vi "Command Rotate Ninety About Tote.vi"(2 "Input Robot System Funtions":T1, 3 "Cmd Parameter 1":dbl, 4 "Cmd Parameter 2":dbl, 5 "Startup":bool) -> (0 "Output Robot System Functions":T1, 1 "Completed":bool=TRUE)   [LabVIEW 2014]
uses:
  Subsystems VIs/Robot Commands.ctl
  Command Execution State.ctl
  Global Variables/Sensor Data (Edited).vi
  Global Variables/Settings.vi
panel:
  in  "Robot Twist Y":dbl=-19.0 format="%#_13g"
  in  "Robot Twist X":dbl=8.0 format="%#_13g"
  out "PID Tracking":cluster{"Goal Wheel Position":dbl, dbl}(graph)={"Goal Wheel Position"=0.0, -90.17571233858979}
  # "Sample robot\ncontrol output.\nReplace with \nactual teleop \ncontrol signal \nstructure."
  # "Field Centric"
  # "Field Centric"
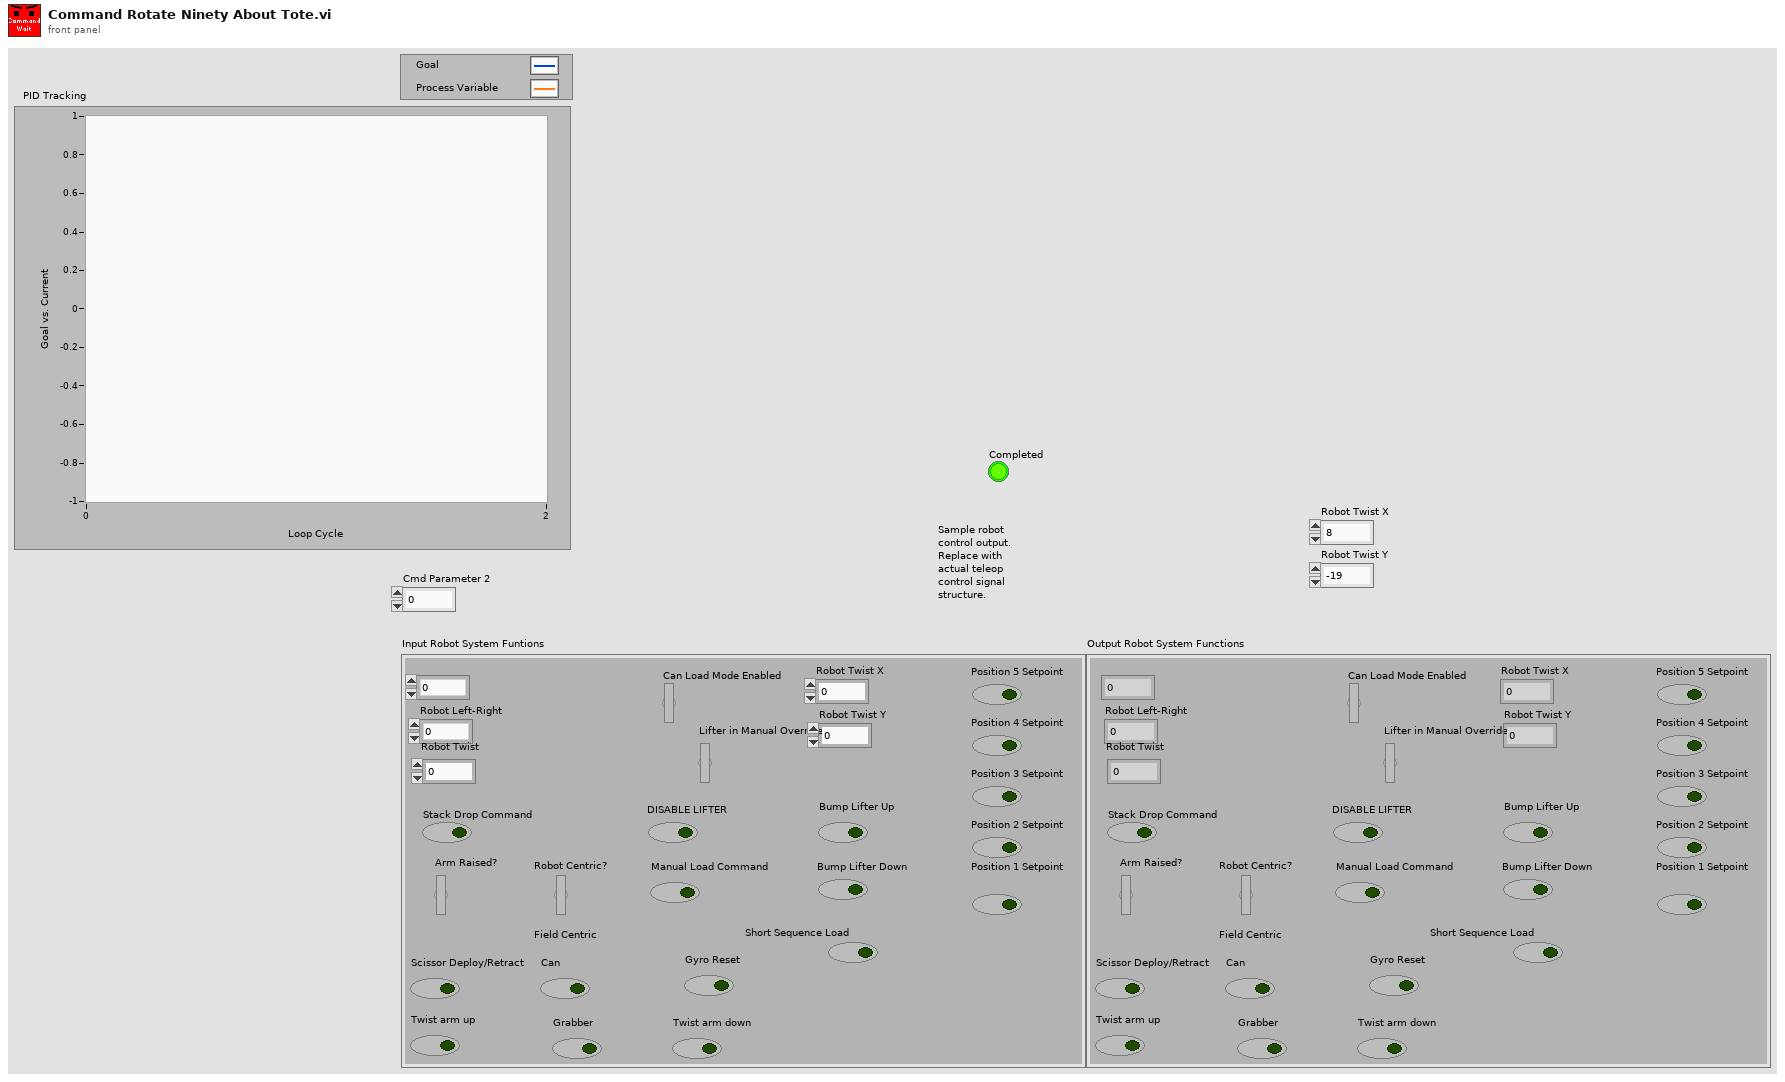
[diagram p1: front panel]
types:
  T1 = typedef "Robot Commands.ctl" = cluster{"Robot Forward-Reverse":dbl, "Robot Left-Right":dbl, "Robot Twist":dbl, "Can Load Mode Enabled":bool, "Lifter in Manual Override?":bool, "Stack Drop Command":bool, "Arm Raised?":bool, "DISABLE LIFTER":bool, "Position 1 Setpoint":bool, "Position 2 Setpoint":bool, "Position 3 Setpoint":bool, "Position 4 Setpoint":bool, "Position 5 Setpoint":bool, "Bump Lifter Down":bool, "Bump Lifter Up":bool, "Manual Load Command":bool, "Robot Centric?":bool, "Scissor Deploy/Retract":bool, "Grabber":bool, "Can":bool, "Twist arm up":bool, "Gyro Reset":bool, "Twist arm down":bool, "Short Sequence Load":bool, "Robot Twist X":dbl, "Robot Twist Y":dbl}
  T2 = typedef "Command Execution State.ctl" = enum16{"Initialize", "Execute", "Finish"}
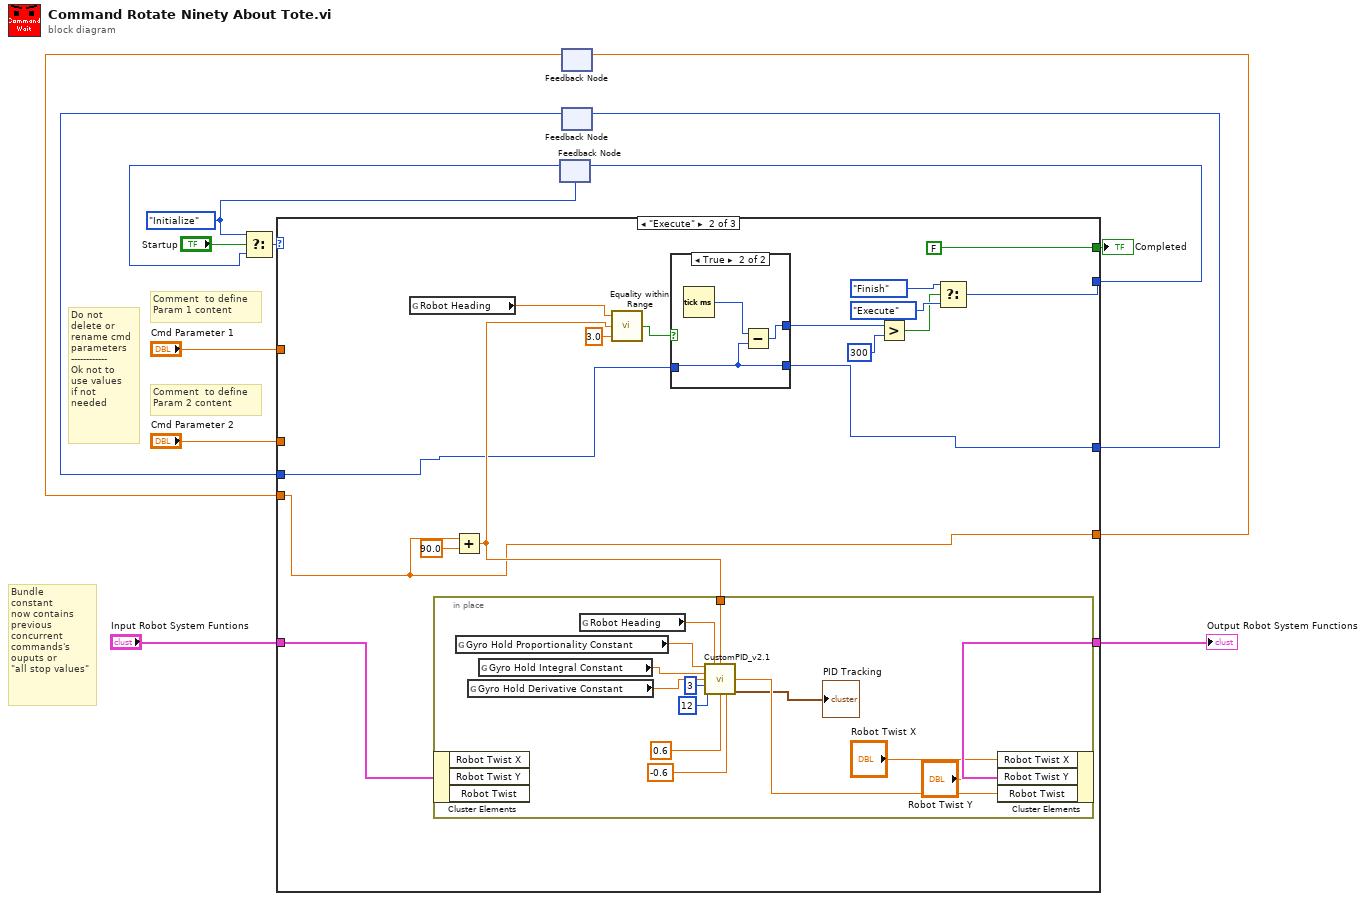
[diagram p0: block diagram]
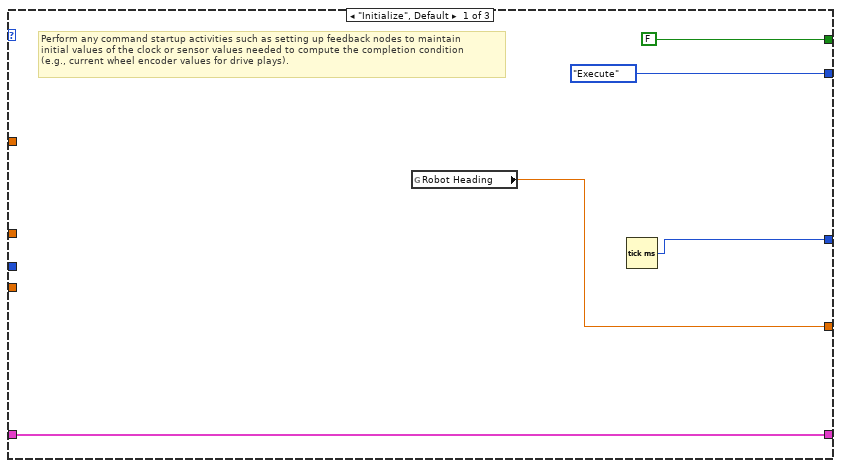
[diagram p2: hidden frame]
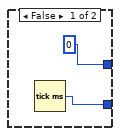
[diagram p3: hidden frame]
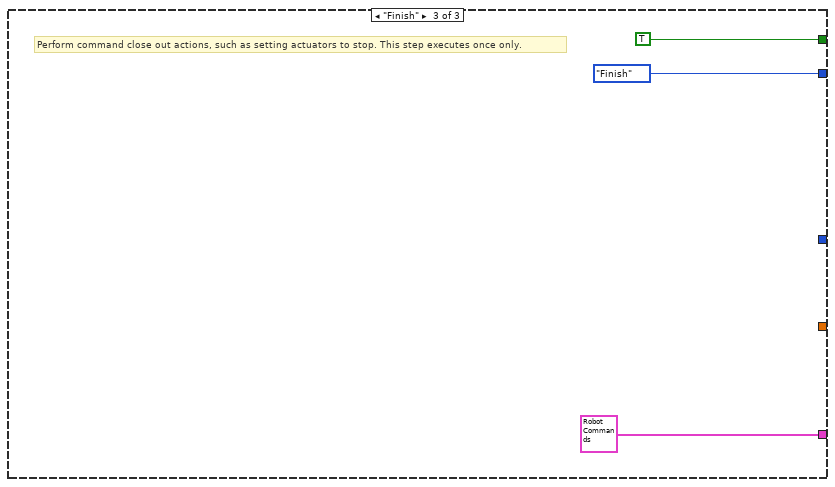
[diagram p4: hidden frame]
diagram:
  w9 = Command_Execution_State."Initialize" ("Play State")
  # "Bundle \nconstant\nnow contains\nprevious \nconcurrent\ncommands's\nouputs or\n\"all stop values\""
  # "Do not \ndelete or\nrename cmd\nparameters\n------------\nOk not to \nuse values\nif not \nneeded"
  # "Comment  to define\nParam 2 content"
  # "Comment  to define\nParam 1 content"
  n1 = feedback #1(w9) -> (w10:T2)
  n2 = Select(t=w9, s="Startup", f=w10) -> (s? t:f=w14:T2)
  n3 = feedback #2() -> (w3:dbl)  [unwired: 1 in]
  n4 = feedback #3() -> (w1:u32)  [unwired: 1 in]
  n5 = case shown="\"Execute\"" w14 {
    tunnel: [FALSE FALSE TRUE] -> w12
    tunnel: [Command_Execution_State."Execute" ("Play State") w21 Command_Execution_State."Finish" ("f")] -> w11
    tunnel: "Cmd Parameter 1" -> [_ _ _]
    tunnel: "Cmd Parameter 2" -> [_ _ _]
    tunnel: [w17 w25 T1 {"Robot Forward-Reverse"=0.0, "Robot Left-Right"=0.0, "Robot Twist"=0.0, "Can Load Mode Enabled"=FALSE, "Lifter in Manual Override?"=FALSE, "Stack Drop Command"=FALSE, "Arm Raised?"=FALSE, "DISABLE LIFTER"=FALSE, "Position 1 Setpoint"=FALSE, "Position 2 Setpoint"=FALSE, "Position 3 Setpoint"=FALSE, "Position 4 Setpoint"=FALSE, "Position 5 Setpoint"=FALSE, "Bump Lifter Down"=FALSE, "Bump Lifter Up"=FALSE, "Manual Load Command"=FALSE, "Robot Centric?"=FALSE, "Scissor Deploy/Retract"=FALSE, "Grabber"=FALSE, "Can"=FALSE, "Twist arm up"=FALSE, "Gyro Reset"=FALSE, "Twist arm down"=FALSE, "Short Sequence Load"=FALSE, "Robot Twist X"=0.0, "Robot Twist Y"=0.0} ("Input Robot System Funtions")] -> w5
    tunnel: "Input Robot System Funtions" -> [w17 w24 _]
    tunnel: [w16 w26 _] -> w4
    tunnel: w3 -> [_ w26 _]
    tunnel: [w15 w23 _] -> w2
    tunnel: w1 -> [_ w22 _]
    frame "Initialize", Default {
      # "Perform any command startup activities such as setting up feedback nodes to maintain \ninitial values of the clock or sensor values needed to compute the completion condition\n(e.g., current wheel encoder values for drive plays)."
      n6 = global read "Sensor Data (Edited).vi" "Robot Heading"() -> (w16:dbl)
      n7 = Tick Count (ms)() -> (millisecond timer value=w15:u32)
    }
    frame "Execute" {
      n8 = global read "Sensor Data (Edited).vi" "Robot Heading"() -> (w34:dbl)
      n9 = Add(x=w26, y=90.0) -> (x+y=w27:dbl)
      n10 = in-place {
        in-place-border: w27 -> [w44]
        n11 = in-place-cluster #4(w24) -> ()  [unwired: 3 out]
        n12 = global read "Settings.vi" "Gyro Hold Proportionality Constant"() -> (w52:dbl)
        n13 = global read "Settings.vi" "Gyro Hold Derivative Constant"() -> (w50:dbl)
        n14 = global read "Settings.vi" "Gyro Hold Integral Constant"() -> (w51:dbl)
        n15 = global read "Sensor Data (Edited).vi" "Robot Heading"() -> (w53:dbl)
        n16 = call "CustomPID_v2.1.vi"("Kp"=w52, "Process Variable"=w53, "Goal"=w44, "Ki"=w51, "Kd"=w50, "N-Diff"=3, "N-Int"=12, "Max Ouput"=0.6, "Min Output"=-0.6) -> ("Command"=w54:dbl, "PID Tracking"=→"PID Tracking":cluster{"Goal Wheel Position":dbl, dbl})  [unwired: 4 in, 1 out]
        n17 = in-place-cluster #4("Robot Twist X"="Robot Twist X", "Robot Twist Y"="Robot Twist Y", "Robot Twist"=w54) -> (w25:T1)
      }
      n18 = call "Equality within Range.vi"("Range"=3.0, "Y"=w27, "X"=w34) -> ("X = Y within Range?"=w33:bool)
      n19 = case shown="True" w33 {
        tunnel: [w37 w40] -> w23
        tunnel: w22 -> [_ w40]
        tunnel: [0 w41] -> w30
        frame False {
          n20 = Tick Count (ms)() -> (millisecond timer value=w37:u32)
        }
        frame True {
          n21 = Tick Count (ms)() -> (millisecond timer value=w39:u32)
          n22 = Subtract(x=w39, y=w40) -> (x-y=w41:u32)
        }
      }
      n23 = Greater?(x=w30, y=u32 300) -> (0:w32:bool)
      n24 = Select(t=Command_Execution_State."Finish" ("Play State"), s=w32, f=Command_Execution_State."Execute" ("Play State")) -> (s? t:f=w21:T2)
    }
    frame "Finish" {
      # "Perform command close out actions, such as setting actuators to stop. This step executes once only."
    }
  }
  "Completed" <- w12
  "Output Robot System Functions" <- w5
  n25 = feedback-in #1(w11) -> ()
  n26 = feedback-in #2(w4) -> ()
  n27 = feedback-in #3(w2) -> ()
